vi "switchboard_channel_mapping.vi"(3 "error in":errorcluster, 5 "Input parameters":T1={"Measurement type"=enum."Debug", "Sensor type"=enum."HPK_8in_271ch", "Identifier"="test.txt", "Open after execution?"=FALSE, "Plot after execution?"=FALSE, "Display channel"=0, "Voltage Delay (s)"=0.5, "Switch Delay (s)"=0.01, "VISA resource name source"="", "VISA resource name DMM"="", "VISA resource name LCR"="", "Compliance  Level (A)"=10.0, "Voltage Limit (V)"=1000.0, "Data storage location"="", "Scan voltages"="", "Use source as DMM?"=FALSE, "LCR signal frequenzy (Hz)"=10.0, "DMM device"=enum."Keithley2001", "Sampling number"=1, "Use env. sensors on"=enum."Sensirion sht1x/7x", "Switchboard Handle"=0, "Use Switchboard"=FALSE, "LCR signal voltage (V)"=10000.0, "Repeat"=1, "Scan voltages IV"="", "Scan voltages CV"="", "Hex pad numbers?"=FALSE, "Set measurement type"=enum."Debug", "Custom pad scan"="", "IV voltage Delay (s)"=0.5, "CV voltage Delay (s)"=0.5, "Needle measurement?"=FALSE, "Comments"="test.txt", "LCR signal frequenzy (kHz)"=10.0, "Compliance  Level (uA)"=10.0, "Open Correction Array"=array2304x3[6912 elements], "Current set voltage"=0.0, "Last set voltage"=0.0, "Current channel"=0, "Last OpenCorrection index"=-1, "Total curr/vltg every x steps"=10, "Current channel iteration"=0, "No CV corrections"=FALSE, "Mapfile"="", "Corrfile"="", "IV voltage file"=path "", "CV voltage file"=path "", "IV Switch Delay (s)"=0.01, "CV Switch Delay (s)"=0.01, "Invert polarity"=FALSE, "Set debug dirs"=FALSE, "Is n on p"=FALSE, "Source interlock?"=TRUE, "Voltage file used?"=FALSE, "Pad mask"="", "Mask pad above (uA)"=1.0, "LCR device"=enum."LCR_E4980", "Source device"=enum."Source_2410", "HexPlot binary path"="", "PadReductionFactor"=1.0, "Temperature degC"="", "Fluence [neq]"="", "Annealing [min]"=""} {"CV Switch Delay (s)" format="%#_13g"; "IV Switch Delay (s)" format="%#_13g"; "Last set voltage" format="%#_13g"; "Current set voltage" format="%#_13g"; "CV voltage Delay (s)" format="%#_13g"; "IV voltage Delay (s)" format="%#_13g"; "Voltage Limit (V)" format="%#_13g"; "Voltage Delay (s)" format="%#_13g"; "Switch Delay (s)" format="%#_13g"}) -> (0 "error out":errorcluster, 1 "Custom pad array":i32[](array[numeric]), 2 "Channel switch array":i32[](array[numeric])=[255, 309, 187, 232, 316, 313, 383, 125, 177, 246, 235, 303, 372, 444, 445, 56, 112, 190, 189, 234, 318, 301, 375, 432, 508, 511, 58, 124, 127, 176, 254, 233, 311, 374, 442, 447, 498, 509, 60, 114, 188, 191, 236, 314, 317, 373, 434, 506, 503, 61, 126, 119, 178, 252, 245, 297, 382, 440, 439, 500, 507, 62, 113, 186, 185, 247, 298, 319, 371, 436, 504, 505, 59, 118, 123, 179, 250, 253, 306, 380, 377, 437, 502, 501, 57, 115, 182, 248, 249, 237, 299, 369, 438, 441, 499, 120, 116, 121, 181, 240, 251, 312, 378, 379, 435, 510, 497, 122, 117, 180, 238, 241, 308, 315, 368, 446, 443, 496, 184, 183, 242, 239, 302, 376, 381, 433, 244, 243, 304, 307, 370, 300, 305, 310, 296, 40, 41, 42, 43, 44, 45, 46, 47, 63, 48, 49, 50, 51, 52, 53, 54, 55])   [LabVIEW 2020]
doc: "Reads the switchboard to probe card map and set corresponding channel list."
uses:
  input_params.ctl
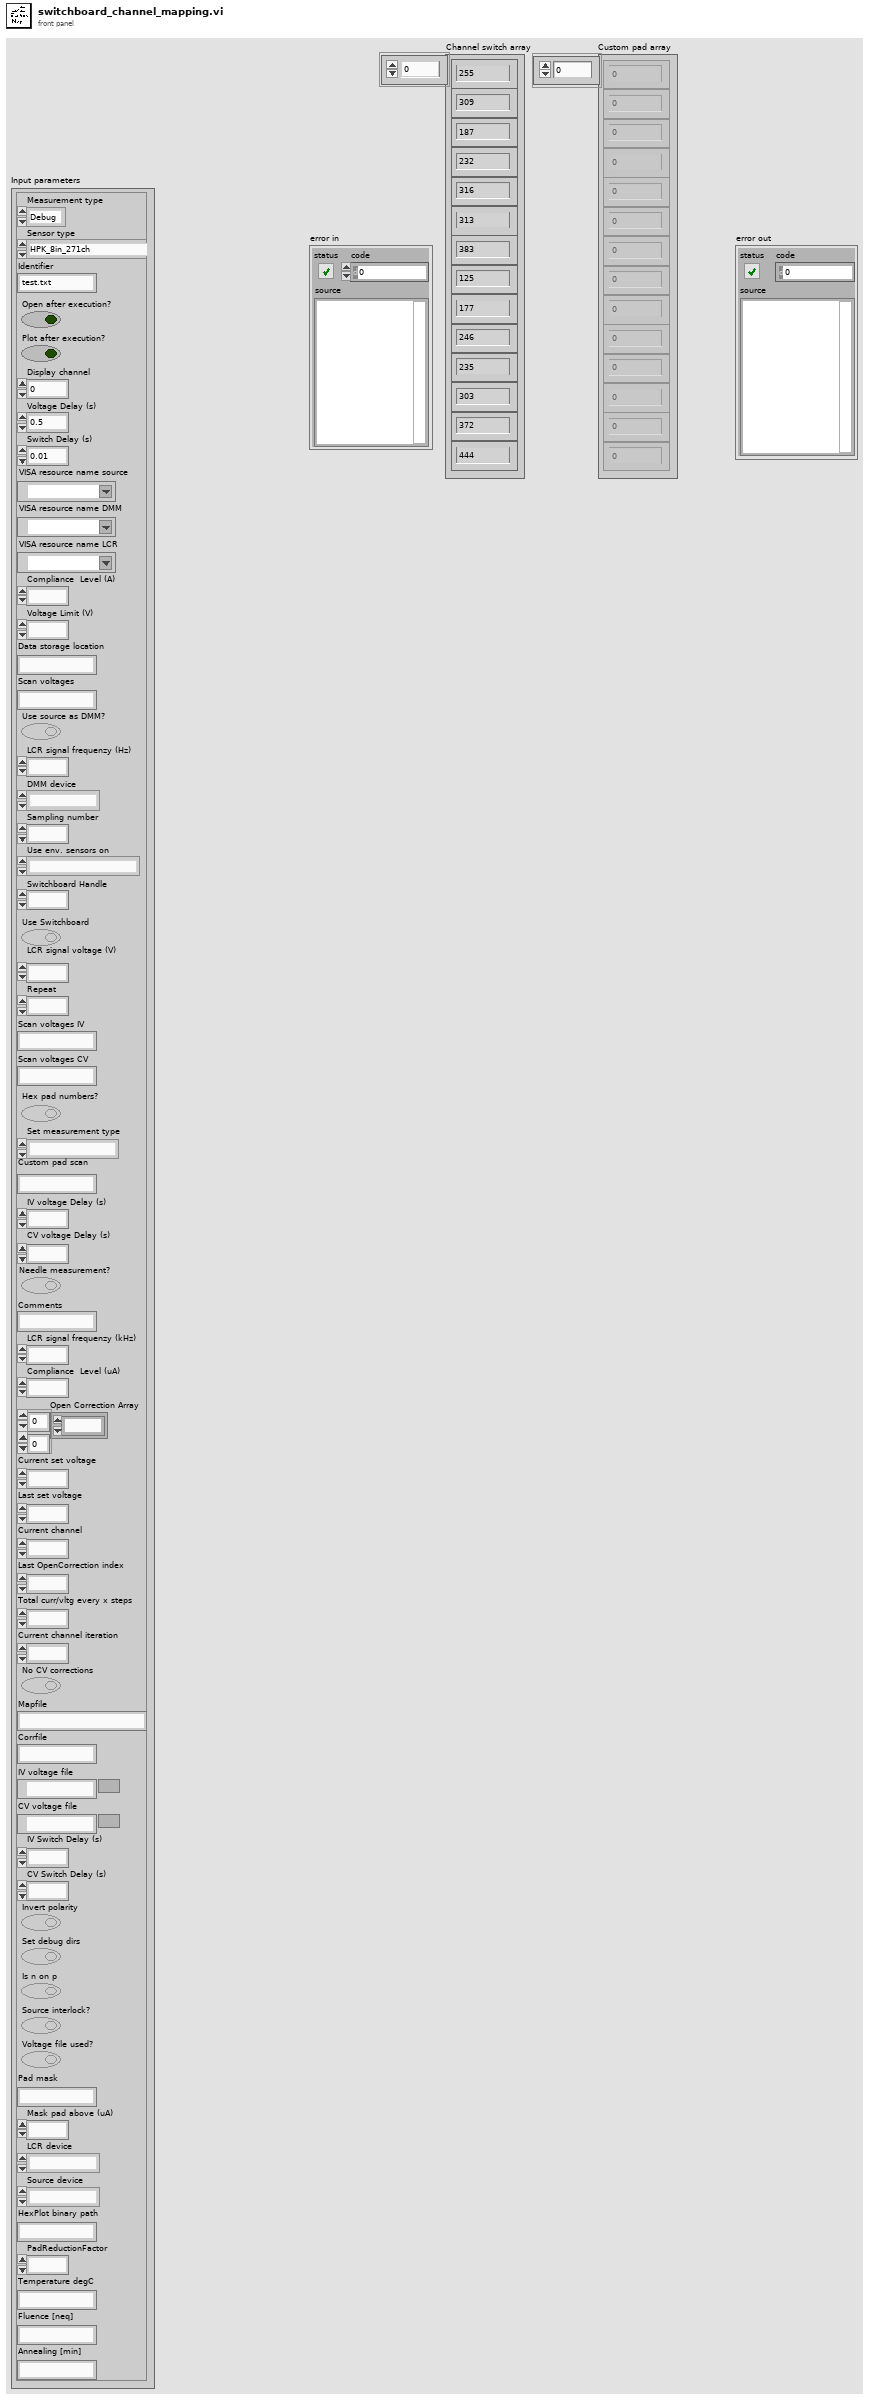
[diagram p1: front panel]
types:
  T1 = typedef "input_params.ctl" = cluster{"Measurement type":enum16{"IV", "CV", "Debug", "Test_contact"}, "Sensor type":enum16{"HPK_6in_135ch", "HPK_8in_271ch", "IFX_8in_256ch", "Diode", "HPK_6in_239ch", "Full_Matrix", "HPK_8in_271ch_full", "LumiCal", "HPK_8in_444ch", "HPK_8in_198ch_2019", "HPK_8in_MGW_LD_full", "HPK_8in_MGW_LD_a_type_top", "HPK_8in_MGW_LD_a_type_bottom", "HPK_8in_MGW_LD_b_type_left", "HPK_8in_MGW_LD_b_type_right", "HPK_8in_MGW_LD_c_type_left", "HPK_8in_MGW_LD_c_type_right", "HPK_8in_MGW_HD_full", "HPK_8in_MGW_HD_a_type_top", "HPK_8in_MGW_HD_a_type_bottom", "HPK_8in_MGW_HD_b_type_left", "HPK_8in_MGW_HD_b_type_right", "HPK_8in_MGW_HD_c_type_left", "HPK_8in_MGW_HD_c_type_right", "CALICE_6in_256ch"}, "Identifier":string, "Open after execution?":bool, "Plot after execution?":bool, "Display channel":i32, "Voltage Delay (s)":dbl, "Switch Delay (s)":dbl, "VISA resource name source":refnum<visa-resource-name>, "VISA resource name DMM":refnum<visa-resource-name>, "VISA resource name LCR":refnum<visa-resource-name>, "Compliance  Level (A)":dbl, "Voltage Limit (V)":dbl, "Data storage location":string, "Scan voltages":string, "Use source as DMM?":bool, "LCR signal frequenzy (Hz)":dbl, "DMM device":enum16{"Keithley2001", "Keithley2450", "Keithley2410", "Keithley6485", "Keithley6487", "Keithley6517"}, "Sampling number":i32, "Use env. sensors on":enum16{"Sensirion sht1x/7x", "Switch Matrix", "Probecard"}, "Switchboard Handle":u32, "Use Switchboard":bool, "LCR signal voltage (V)":dbl, "Repeat":i32, "Scan voltages IV":string, "Scan voltages CV":string, "Hex pad numbers?":bool, "Set measurement type":enum16{"IV", "CV", "Debug", "Test_contact", "IV+CV"}, "Custom pad scan":string, "IV voltage Delay (s)":dbl, "CV voltage Delay (s)":dbl, "Needle measurement?":bool, "Comments":string, "LCR signal frequenzy (kHz)":dbl, "Compliance  Level (uA)":dbl, "Open Correction Array":dbl[][], "Current set voltage":dbl, "Last set voltage":dbl, "Current channel":i32, "Last OpenCorrection index":i32, "Total curr/vltg every x steps":i32, "Current channel iteration":i32, "No CV corrections":bool, "Mapfile":string, "Corrfile":string, "IV voltage file":path, "CV voltage file":path, "IV Switch Delay (s)":dbl, "CV Switch Delay (s)":dbl, "Invert polarity":bool, "Set debug dirs":bool, "Is n on p":bool, "Source interlock?":bool, "Voltage file used?":bool, "Pad mask":string, "Mask pad above (uA)":dbl, "LCR device":enum16{"LCR_E4980", "AGILENT_4263X"}, "Source device":enum16{"Source_2410", "Source_6487"}, "HexPlot binary path":string, "PadReductionFactor":dbl, "Temperature degC":string, "Fluence [neq]":string, "Annealing [min]":string}
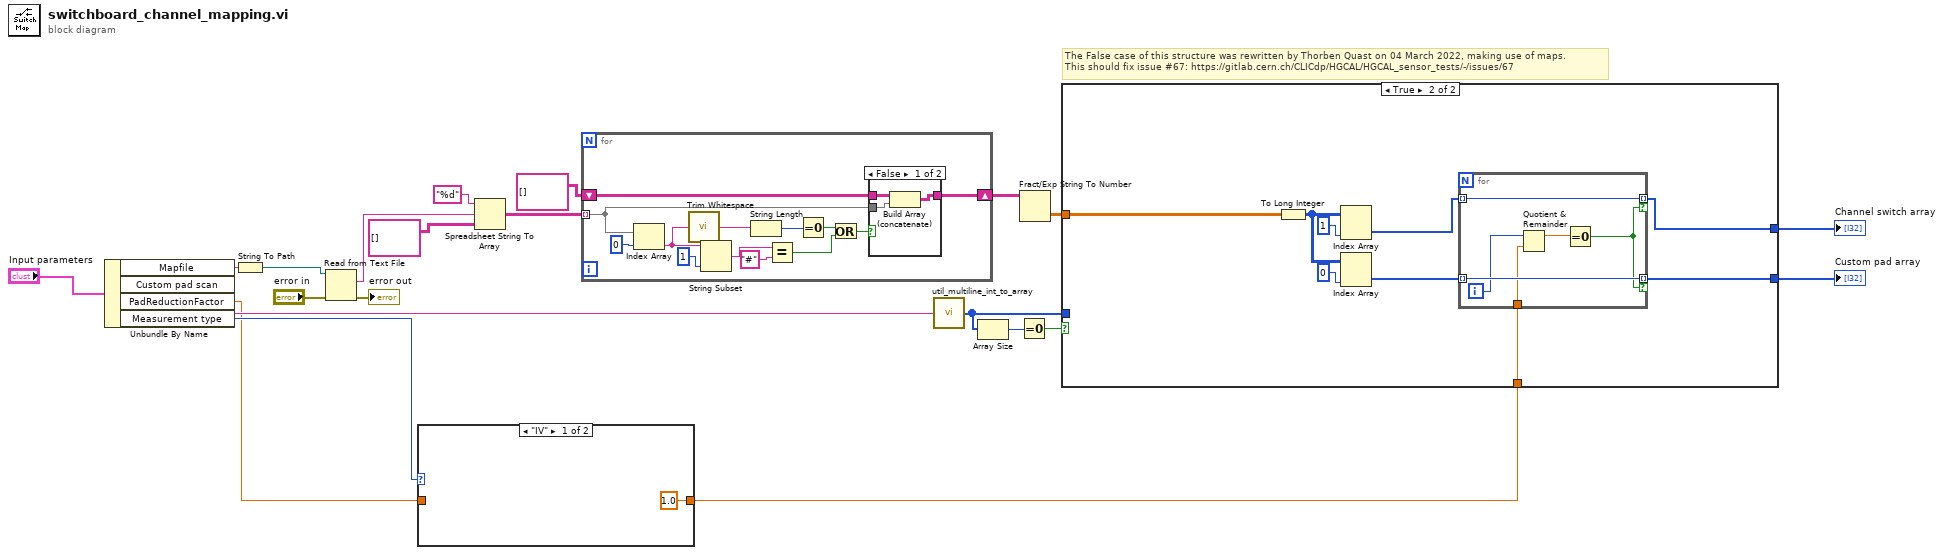
[diagram p0: block diagram]
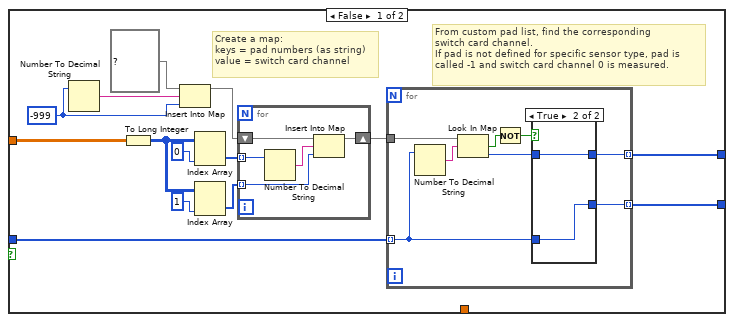
[diagram p4: hidden frame]
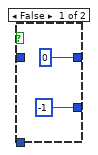
[diagram p5: hidden frame]
diagram:
  # "The False case of this structure was rewritten by Thorben Quast on 04 March 2022, making use of maps.\nThis should fix issue #67: https://gitlab.cern.ch/CLICdp/HGCAL/HGCAL_sensor_tests/-/issues/67"
  n1 = Unbundle By Name("Input parameters") -> ("Mapfile"=w14:string, "Custom pad scan"=w20:string, "PadReductionFactor"=w1:dbl, "Measurement type"=w3:enum16{"IV", "CV", "Debug", "Test_contact"})
  n2 = String To Path(string=w14) -> (path=w6:path)
  n3 = Read from Text File(file (use dialog)=w6, error in="error in") -> (text=w7:string, error out=→"error out":errorcluster)  [unwired: 2 in, 2 out]
  n4 = case shown="\"IV\"" w3 {
    tunnel: [1.0 ("PadReductionFactor") w23] -> w2
    tunnel: w1 -> [_ w23]
    frame "IV" {
    }
    frame Default {
    }
  }
  n5 = Spreadsheet String To Array(format string="%d", spreadsheet string=w7, array type (2D Dbl)=string[][] [] ("Array")) -> (array=w5:string[][])  [unwired: 1 in]
  n6 = for {
    shift-right: [w27] -> w11
    shift-left: string[][] [] ("subarray") -> [w28]
    tunnel: w5 -> [w25] mode=indexing
    n7 = Index Array(array=w25, index=0 ("index (row)")) -> (element=w26:string)
    n8 = call <vilib>:"Trim Whitespace.vi"("string"=w26) -> ("trimmed string"=w32:string)  [unwired: 1 in]
    n9 = String Subset(string=w26, length (rest)=1 ("length (rest)")) -> (substring=w35:string)  [unwired: 1 in]
    n10 = String Length(string=w32) -> (length=w33:i32)
    n11 = Equal?(x=w35, y="#") -> (x = y?=w30:bool)
    n12 = Equal To 0?(x=w33) -> (x = 0?=w31:bool)
    n13 = Or(x=w31, y=w30) -> (x .or. y?=w29:bool)
    n14 = case shown="False" w29 {
      tunnel: w28 -> [w39 w40]
      tunnel: [w38 w40] -> w27
      tunnel: w25 -> [w37 _]
      frame False {
        n15 = Build Array (concatenate)(w39, w37) -> (w38:string[][])
      }
      frame True {
      }
    }
  }
  n16 = call "util_multiline_int_to_array.vi"("Multiline integer string"=w20) -> ("Array"=w17:i32[])
  n17 = Array Size(array=w17) -> (size(s)=w16:i32)
  n18 = Equal To 0?(x=w16) -> (x = 0?=w15:bool)
  n19 = Fract/Exp String To Number(string=w11) -> (number=w4:dbl[][])  [unwired: 3 in, 1 out]
  n20 = case shown="True" w15 {
    tunnel: w17 -> [w50 _]
    tunnel: [w42 w75] -> w19
    tunnel: [w41 w74] -> w18
    tunnel: w4 -> [w51 w77]
    tunnel: w2 -> [_ w72]
    frame False {
      w47 = -999
      # "From custom pad list, find the corresponding\nswitch card channel.\nIf pad is not defined for specific sensor type, pad is \ncalled -1 and switch card channel 0 is measured."
      # "Create a map:\nkeys = pad numbers (as string)\nvalue = switch card channel"
      n21 = Number To Decimal String(number=w47) -> (decimal integer string=w48:string)  [unwired: 1 in]
      n22 = To Long Integer(number=w51) -> (32bit integer=w52:i32[][])
      n23 = Insert Into Map(map in=map{string, i32} {}, key=w48, value=w47) -> (map out=w44:map{string, i32})  [unwired: 2 out]
      n24 = Index Array(array=w52, index (col)=0) -> (element=w45:i32[])  [unwired: 1 in]
      n25 = Index Array(array=w52, index (col)=1) -> (element=w46:i32[])  [unwired: 1 in]
      n26 = for {
        tunnel: w46 -> [w59] mode=indexing
        tunnel: w45 -> [w58] mode=indexing
        shift-right: [w56] -> w43
        shift-left: w44 -> [w55]
        n27 = Number To Decimal String(number=w58) -> (decimal integer string=w57:string)  [unwired: 1 in]
        n28 = Insert Into Map(map in=w55, key=w57, value=w59) -> (map out=w56:map{string, i32})  [unwired: 2 out]
      }
      n29 = for {
        tunnel: w50 -> [w61] mode=indexing
        tunnel: w43 -> [w67]
        tunnel: [w60] -> w41 mode=indexing
        tunnel: [w62] -> w42 mode=indexing
        n30 = Number To Decimal String(number=w61) -> (decimal integer string=w66:string)  [unwired: 1 in]
        n31 = Look In Map(map=w67, key=w66) -> (key not found?=w64:bool, value=w63:i32)  [unwired: 1 in]
        n32 = Not(x=w64) -> (.not. x?=w65:bool)
        n33 = case shown="True" w65 {
          tunnel: [0 ("value") w71] -> w62
          tunnel: w63 -> [_ w71]
          tunnel: w61 -> [_ w70]
          tunnel: [-1 ("Numeric Control") w70] -> w60
          frame False {
          }
          frame True {
          }
        }
      }
    }
    frame True {
      n34 = To Long Integer(number=w77) -> (32bit integer=w78:i32[][])
      n35 = Index Array(array=w78, index (col)=1 ("disabled index (col)")) -> (element=w76:i32[])  [unwired: 1 in]
      n36 = Index Array(array=w78, index (col)=0) -> (element=w73:i32[])  [unwired: 1 in]
      n37 = for {
        tunnel: w76 -> [w86] mode=indexing
        tunnel: [w86] -> w75 mode=indexing if=w83
        tunnel: [w85] -> w74 mode=indexing if=w83
        tunnel: w73 -> [w85] mode=indexing
        tunnel: w72 -> [w81]
        i -> [w82]
        n38 = Quotient & Remainder(x=w82, y=w81) -> (x-y*floor(x/y)=w84:dbl)  [unwired: 1 out]
        n39 = Equal To 0?(x=w84) -> (x = 0?=w83:bool)
      }
    }
  }
  "Channel switch array" <- w19
  "Custom pad array" <- w18
